vi "Change CH Name.vi"(8 "error in (no error)":errorcluster, 9 "Old #":i32, 10 "New #":i32, 11 "Node Ptr":T1 format="%.0x") -> (0 "error out":errorcluster, 3 "Node Ptr out":T1 format="%.0x")   [LabVIEW 2021, in "NI 272x Resistive Simulation Custom Device Configuration.lvlib"]
uses:
  NI 272x Resistive Simulation Custom Device Configuration.lvlib
  Program Files/National Instruments/LabVIEW 2021/vi.lib/NI VeriStand/Custom Device API/Custom Device Item Ref.ctl
  Program Files/National Instruments/LabVIEW 2021/vi.lib/NI VeriStand/Custom Device API/Custom Device API.lvlib
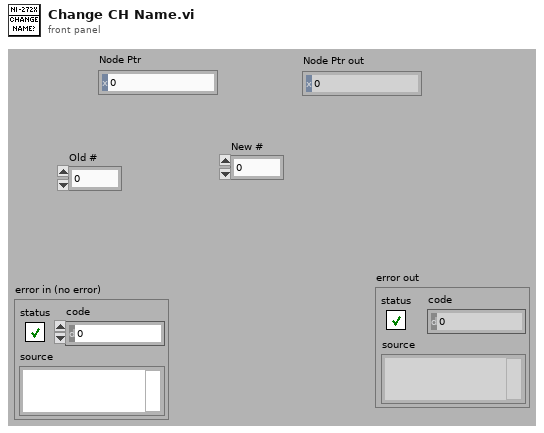
[diagram p1: front panel]
types:
  T1 = typedef "Custom Device API.lvlib/Custom Device Item Ref.ctl" = u64
  T2 = typedef "Custom Device API.lvlib/Custom Device Item Info.ctl" = cluster{"Name":string, "Is Channel":bool, "GUID":string, "Is Waveform":bool}
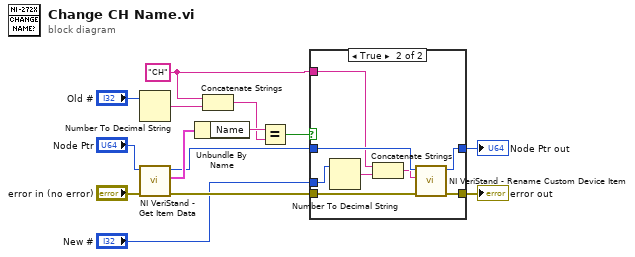
[diagram p0: block diagram]
diagram:
  w1 = "CH" ("string")
  n1 = Number To Decimal String(number="Old #") -> (decimal integer string=w11:string)  [unwired: 1 in]
  n2 = call "NI VeriStand - Get Item Data.vi"("error in (no error)"="error in (no error)", "Item Ref in"="Node Ptr") -> ("error out"=w8:errorcluster, "Item Info"=w13:T2, "Item Ref out"=w7:T1)  [unwired: 7 out]
  n3 = Unbundle By Name(w13) -> ("Name"=w10:string)
  n4 = Concatenate Strings(w1, w11) -> (w9:string)
  n5 = Equal?(x=w10, y=w9) -> (x = y?=w4:bool)
  n6 = case shown="True" w4 {
    tunnel: w8 -> [w16 w24]
    tunnel: w7 -> [w15 w23]
    tunnel: [w15 w22] -> w6
    tunnel: [w16 w21] -> w5
    tunnel: "New #" -> [_ w18]
    tunnel: w1 -> [_ w17]
    frame False {
    }
    frame True {
      n7 = Number To Decimal String(number=w18) -> (decimal integer string=w20:string)  [unwired: 1 in]
      n8 = Concatenate Strings(w17, w20) -> (w19:string)
      n9 = call "NI VeriStand - Rename Custom Device Item.vi"("error in (no error)"=w24, "New Name"=w19, "Item Ref in"=w23) -> ("error out"=w21:errorcluster, "Item Ref out"=w22:T1)  [unwired: 1 in, 6 out]
    }
  }
  "error out" <- w5
  "Node Ptr out" <- w6
